vi "Detector Simulator Generate Image.vi"(11 "samples":i32=4096) -> (3 "image":dbl[][](graph))   [LabVIEW 2020]
uses:
  <vilib>/Analysis/1siggen.llb/General Periodic Sinc.vi
  <vilib>/Analysis/NI_AALBase.lvlib
panel:
  out "Waveform Graph":dbl[](graph)
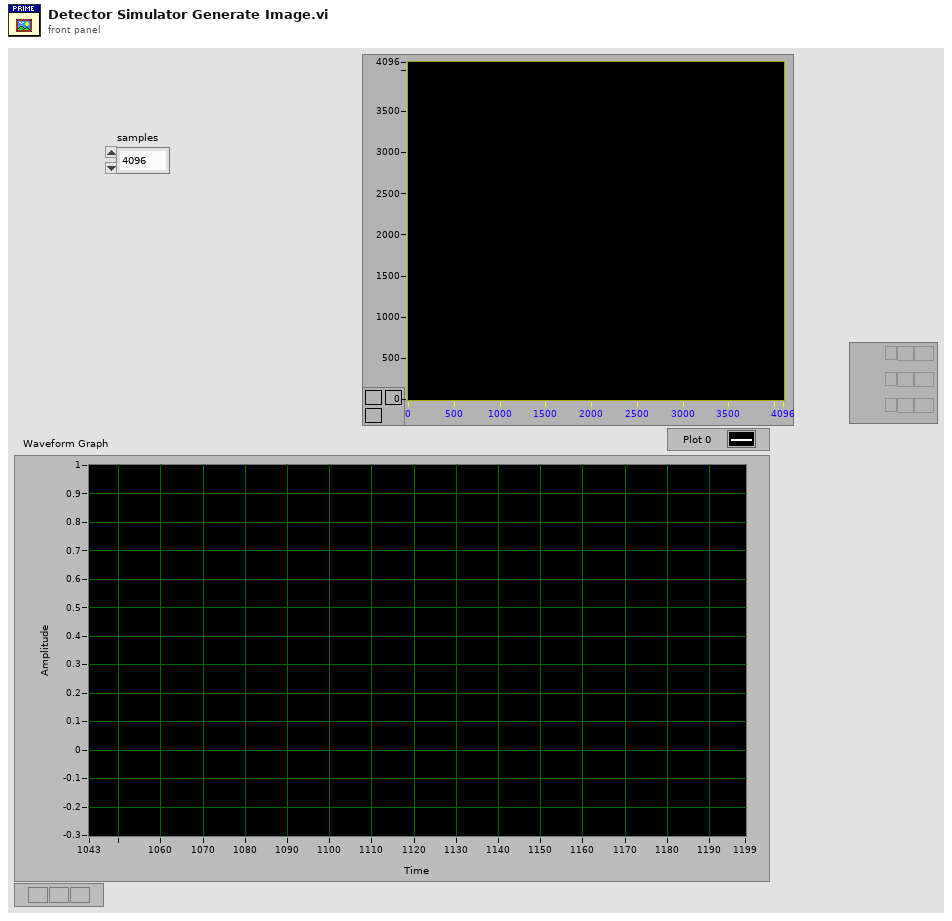
[diagram p1: front panel]
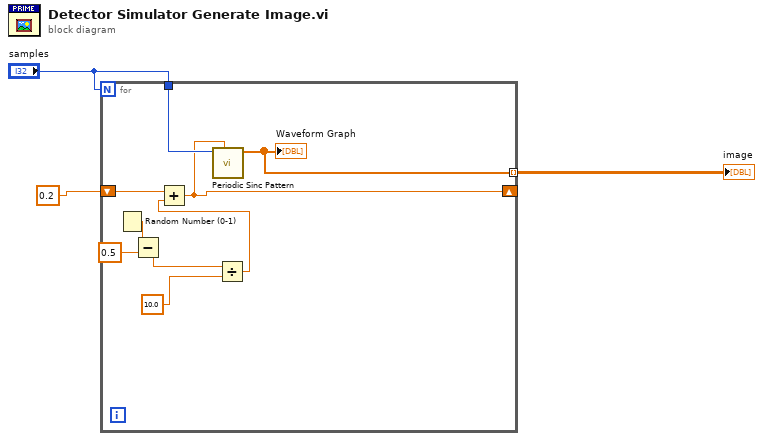
[diagram p0: block diagram]
diagram:
  n1 = for {
    N: "samples" -> [_]
    tunnel: "samples" -> [w12]
    shift-right: [w5] -> _
    shift-left: 0.2 ("delta t (s)") -> [w11]
    tunnel: [w4] -> w1 mode=indexing
    n2 = Random Number (0-1)() -> (number: 0 to 1=w10:dbl)
    n3 = Subtract(x=w10, y=0.5) -> (x-y=w8:dbl)
    n4 = Divide(x=w8, y=10.0) -> (x/y=w6:dbl)
    n5 = Add(x=w11, y=w6) -> (x+y=w5:dbl)
    n6 = call <vilib>:"Periodic Sinc Pattern.vi"("delay (s)"=w5, "samples"=w12) -> ("Periodic Sinc Pattern"=w4:dbl[])  [unwired: 8 in, 1 out]
    "Waveform Graph" <- w4
  }
  "image" <- w1
